vi "Sequence Start.vi"(8 "error in (no error)":errorcluster, 11 "CAP-USB-1 in":refnum<class "CAP-USB-1.lvclass">) -> (0 "error out":errorcluster, 3 "CAP-USB-1 out":refnum<class "CAP-USB-1.lvclass">)   [LabVIEW 2014, in "CAP-USB-1.lvlib" / "CAP-USB-1.lvclass"]
doc: "Envia el comando para comenzar la adquisicion de datos en modo sequence"
uses:
  CAP-USB-1.lvclass
  CAP-USB-1.lvclass/CAP-USB-1.ctl
  API/CAP-USB/CAP-USB.lvlib
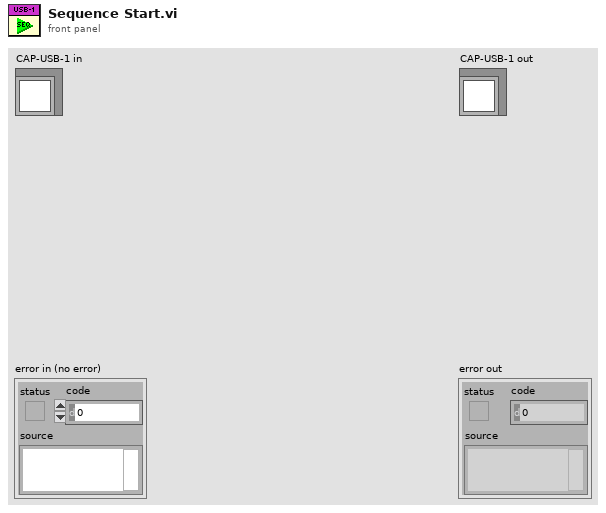
[diagram p1: front panel]
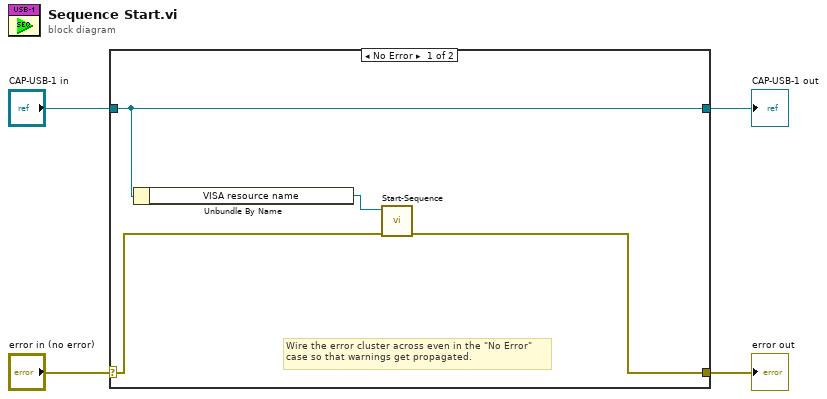
[diagram p0: block diagram]
diagram:
  n1 = case shown="No Error" "error in (no error)" {
    selector: "error in (no error)" -> [w5 w10]
    tunnel: [w6 w10] -> w1
    tunnel: [w8 w9] -> w2
    tunnel: "CAP-USB-1 in" -> [w8 w9]
    frame No Error {
      # "Wire the error cluster across even in the \"No Error\"\ncase so that warnings get propagated."
      n2 = Unbundle By Name(w8) -> ("VISA resource name"=w7:refnum<visa-resource-name>)
      n3 = call "Start-Sequence.vi"("error in (no error)"=w5, "VISA resource name"=w7) -> ("error out"=w6:errorcluster)  [unwired: 8 in, 1 out]
    }
    frame Error {
    }
  }
  "error out" <- w1
  "CAP-USB-1 out" <- w2
